vi "Load_HMI.vi"(8 "error in (no error)":errorcluster caption="entrée d'erreur (pas d'erreur)", 11 "Class Popup (Default) en entrée":refnum<class "Class Popup (Main).lvclass">) -> (0 "error out":errorcluster caption="sortie d'erreur", 3 "Class Popup (Default) en sortie":refnum<class "Class Popup (Main).lvclass">)   [LabVIEW 2020, in "Library Instrument & Equipement.lvlib" / "Library Popup.lvlib" / "Class Popup (Main).lvclass"]
uses:
  Class Popup (Main).lvclass
  Class Popup (Main).lvclass/Class Popup (Main).ctl
  Virtual Launch HMI.vi
  Commun VI/Library Commun.lvlib
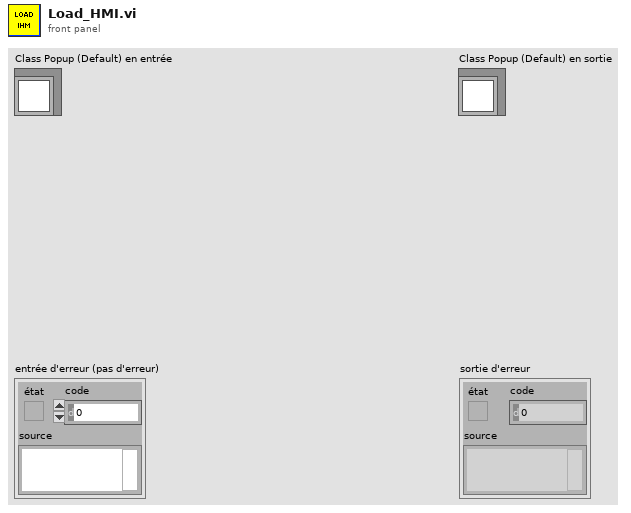
[diagram p1: front panel]
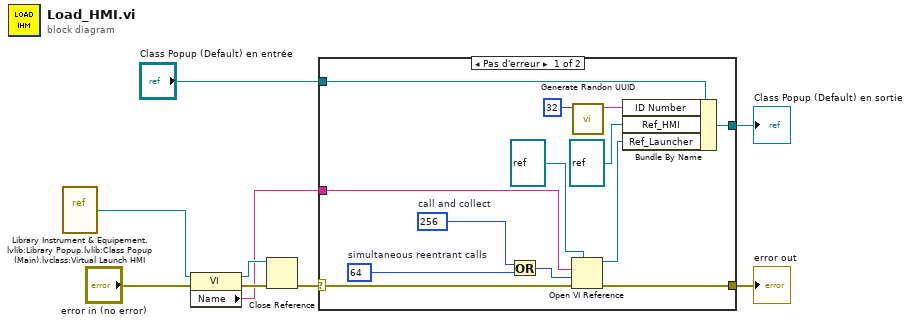
[diagram p0: block diagram]
diagram:
  n1 = vi-ref "Library Instrument & Equipement.lvlib:Library Popup.lvlib:Class Popup (Main).lvclass:Virtual Launch HMI.vi"() -> (w6:refnum<vi>)
  n2 = property class="VI"(reference=w6, error in="error in (no error)") -> (reference out=w5:refnum<vi>, error out=w4:errorcluster, "Name"=w3:string)
  n3 = Close Reference(reference=w5, error in (no error)=w4) -> (error out=w1:errorcluster)
  n4 = case shown="Pas d'erreur" w1 {
    selector: w1 -> [w19 w24]
    tunnel: [w18 w24] -> w9
    tunnel: [w21 w23] -> w8
    tunnel: "Class Popup (Default) en entrée" -> [w22 w23]
    tunnel: w3 -> [w17 _]
    frame No Error {
      w16 = 64  # simultaneous reentrant calls
      w15 = 256  # call and collect
      n5 = Or(x=w15, y=w16) -> (x .or. y?=w14:i32)
      n6 = Open VI Reference(type specifier VI Refnum (for type only)=refnum<vi> refnum ("spécificateur de type du refnum de VI (pour type seulement)"), vi path=w17, options=w14, error in (no error)=w19) -> (vi reference=w10:refnum<vi>, error out=w18:errorcluster)  [unwired: 2 in]
      n7 = call "Generate Randon UUID.vi"("Taille"=32) -> ("chaîne"=w12:string)  [unwired: 10 in]
      n8 = Bundle By Name(cluster=w22, "ID Number"=w12, "Ref_HMI"=refnum<vi> refnum, "Ref_Launcher"=w10) -> (w21:refnum<class "Class Popup (Main).lvclass">)
    }
    frame Error {
    }
  }
  "error out" <- w9
  "Class Popup (Default) en sortie" <- w8
